vi "read.vi"(8 "Error in":errorcluster, 10 "timeout (ms)":i32=500, 11 "EMTestCWS500N.lvclass":refnum<class "EMTestCWS500N.lvclass">) -> (0 "Error Out":errorcluster, 2 "Return String":string, 3 "EMTestCWS500N.lvclass 2":refnum<class "EMTestCWS500N.lvclass">)   [LabVIEW 2013]
uses:
  classes/Devices/emTestCWS500N/EMTestCWS500N.lvclass
panel:
  out "VISA resource name out":refnum<visa-resource-name>
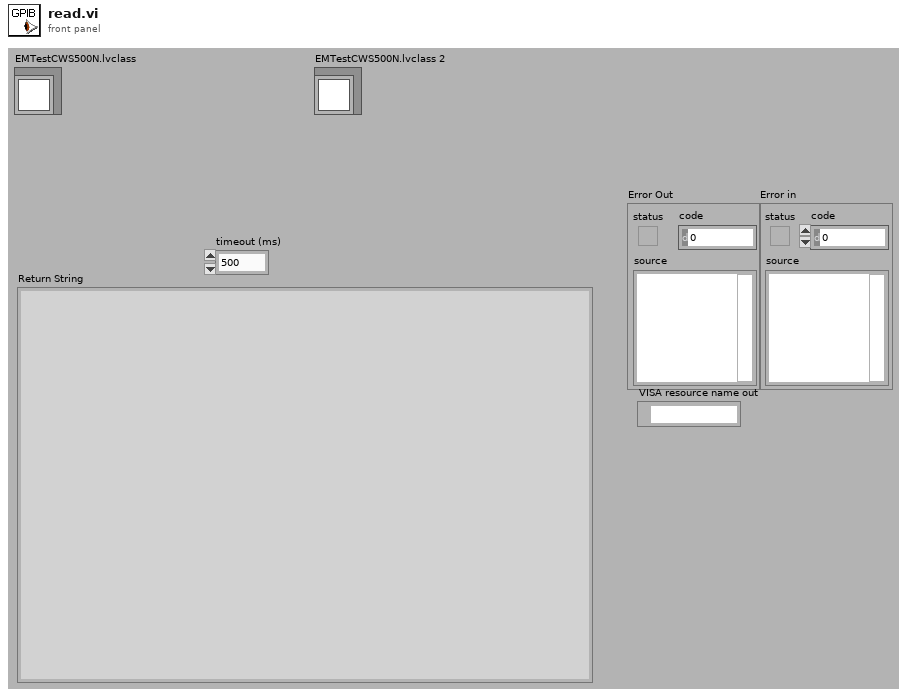
[diagram p1: front panel]
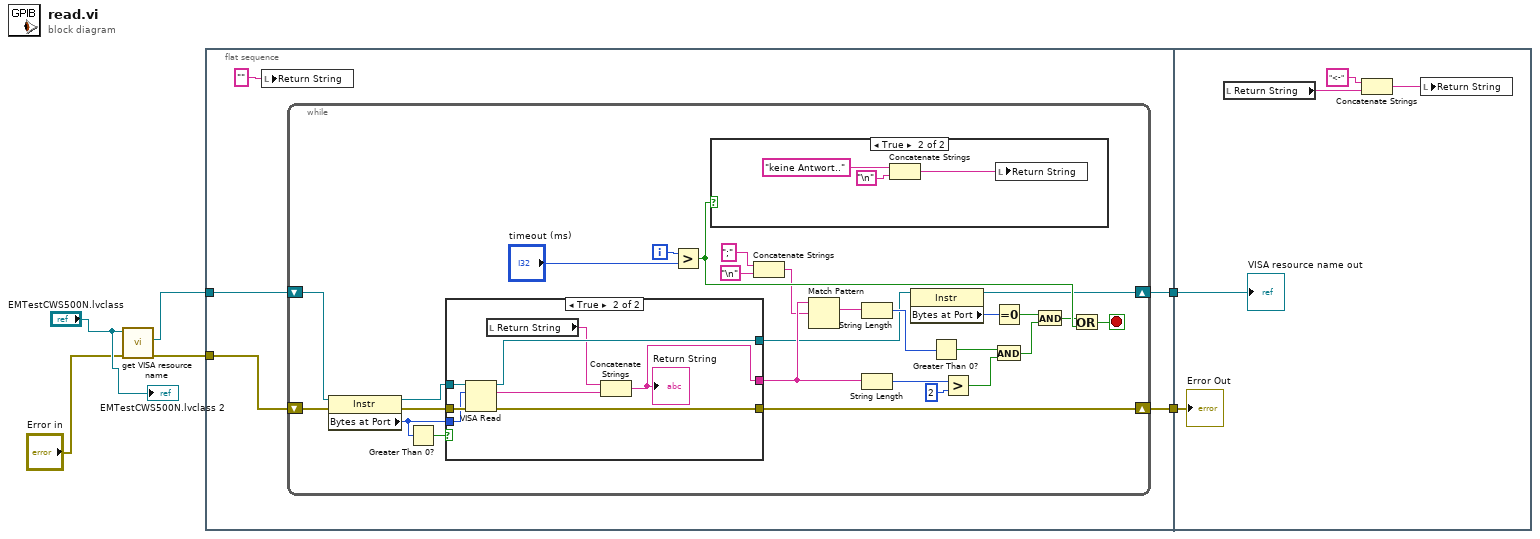
[diagram p0: block diagram]
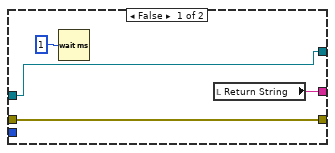
[diagram p3: hidden frame]
diagram:
  n1 = call-dynamic "get VISA resource name.vi"("error in (no error)"="Error in", "DeviceInterface in"="EMTestCWS500N.lvclass") -> ("error out"=w1:errorcluster, "VISA resource name"=w3:refnum<visa-resource-name>)  [unwired: 7 in, 1 out]
  n2 = flat-sequence {
    tunnel: [w11] -> w6
    tunnel: [w10] -> w5
    tunnel: w3 -> [w8]
    tunnel: w1 -> [w7]
    tunnel: w6 -> [w54]
    tunnel: w5 -> [w58]
    frame #0 {
      n3 = local write "Return String"("") -> ()
      n4 = while {
        shift-right: [w20] -> w10
        shift-left: w8 -> [w38]
        shift-right: [w28] -> w11
        shift-left: w7 -> [w35]
        i -> [w33]
        stop <- w31 stop-if-true
        n5 = property class="Instr"(reference=w38, error in=w35) -> (reference out=w37:refnum<visa-resource-name>, error out=w36:errorcluster, "Bytes at Port"=w34:u32)
        n6 = Greater Than 0?(x=w34) -> (x > 0?=w32:bool)
        n7 = case shown="True" w32 {
          tunnel: [w44 w53] -> w28
          tunnel: [w45 w52] -> w21
          tunnel: w37 -> [w45 w51]
          tunnel: w36 -> [w44 w50]
          tunnel: w34 -> [_ w47]
          tunnel: [w42 w46] -> w27
          frame False {
            n8 = Wait (ms)(milliseconds to wait=u32 1) -> ()  [unwired: 1 out]
            n9 = local read "Return String"() -> (w42:string)
          }
          frame True {
            n10 = VISA Read(VISA resource name=w51, byte count=w47, error in (no error)=w50) -> (VISA resource name out=w52:refnum<visa-resource-name>, read buffer=w49:string, error out=w53:errorcluster)  [unwired: 1 out]
            n11 = local read "Return String"() -> (w48:string)
            n12 = Concatenate Strings(w48, w49) -> (w46:string)
            "Return String" <- w46
          }
        }
        n13 = Greater?(x=w33, y="timeout (ms)") -> (0:w30:bool)
        n14 = case shown="True" w30 {
          frame False {
          }
          frame True {
            n15 = Concatenate Strings("keine Antwort.." ("Return String"), "\n") -> (w39:string)
            n16 = local write "Return String"(w39) -> ()
          }
        }
        n17 = Concatenate Strings(";" ("regular expression"), "\n") -> (w13:string)
        n18 = Match Pattern(string=w27, regular expression=w13) -> (match substring=w29:string)  [unwired: 1 in, 3 out]
        n19 = String Length(string=w29) -> (length=w24:i32)
        n20 = String Length(string=w27) -> (length=w26:i32)
        n21 = property class="Instr"(reference=w21) -> (reference out=w20:refnum<visa-resource-name>, "Bytes at Port"=w18:u32)  [unwired: 1 in, 1 out]
        n22 = Greater Than 0?(x=w24) -> (x > 0?=w23:bool)
        n23 = Greater?(x=w26, y=2) -> (0:w22:bool)
        n24 = Equal To 0?(x=w18) -> (x = 0?=w19:bool)
        n25 = And(x=w23, y=w22) -> (x .and. y?=w17:bool)
        n26 = And(x=w19, y=w17) -> (x .and. y?=w16:bool)
        n27 = Or(x=w16, y=w30) -> (x .or. y?=w31:bool)
      }
    }
    frame #1 {
      n28 = local read "Return String"() -> (w55:string)
      n29 = Concatenate Strings("<-" ("string"), w55) -> (w56:string)
      n30 = local write "Return String"(w56) -> ()
      "Error Out" <- w54
      "VISA resource name out" <- w58
    }
  }
  "EMTestCWS500N.lvclass 2" <- "EMTestCWS500N.lvclass"
